vi "reward_behavior_michelle_visjitter_conswin_entice.vi"() -> ()   [LabVIEW 2019]
doc: "The myRIO Project template acquires acceleration data from the onboard accelerometer and displays the changes of acceleration values in a waveform chart."
uses:
  <vilib>/Analysis/Matrix/Datatypes/RealMatrix.ctl
  <vilib>/myRIO/Common/Instrument Driver Framework/myRIO v1.0/Encoder/typedefs/Encoder Signal Mode.ctl
  <vilib>/myRIO/Instrument Drivers/Onboard IO/Encoder/typedefs/Encoder Reference.ctl
  <vilib>/myRIO/Common/Instrument Driver Framework/Utilities/typedefs/myRIO Generic Hardware Reference.ctl
  <vilib>/myRIO/Common/Instrument Driver Framework/Utilities/typedefs/Hardware Version Enum.ctl
  <vilib>/myRIO/Common/Instrument Driver Framework/Utilities/typedefs/myRIO v1.0 Reference.ctl
  <vilib>/myRIO/Common/Instrument Driver Framework/Utilities/typedefs/Generic FPGA Reference.ctl
  <vilib>/myRIO/Common/Instrument Driver Framework/myRIO v1.0/Encoder/typedefs/Encoder Channels Enum.ctl
  <vilib>/myRIO/Common/Instrument Driver Framework/myRIO v1.0/Encoder/typedefs/Encoder Configuration v1.0.ctl
  <vilib>/userdefined/High Color/nirio_resource_hc.ctl
  <vilib>/myRIO/Instrument Drivers/Onboard IO/DIO/typedefs/DIO Reference.ctl
  <vilib>/myRIO/Common/Instrument Driver Framework/myRIO v1.0/DIO/typedefs/DIO Channels List.ctl
  <vilib>/myRIO/Common/Instrument Driver Framework/myRIO v1.0/DIO/typedefs/DIO Channels Enum.ctl
  <vilib>/myRIO/Common/Instrument Driver Framework/Utilities/vis/Is FPGA Ref Available.vi
  <vilib>/myRIO/Common/Instrument Driver Framework/myRIO v1.0/Encoder/vis/myRIO v1.1 Open Encoder.vi
  <vilib>/myRIO/Instrument Drivers/Onboard IO/Encoder/vis/Read.vi
  <vilib>/myRIO/Common/Instrument Driver Framework/myRIO v1.0/DIO/vis/myRIO v1.1 Open DIO.vi
  <vilib>/myRIO/Instrument Drivers/Onboard IO/DIO/vis/Write.vi
  <vilib>/myRIO/Instrument Drivers/Onboard IO/DIO/vis/Read.vi
  <vilib>/myRIO/Common/Instrument Driver Framework/Utilities/vis/Validate Channels.vi
  <vilib>/myRIO/Common/Instrument Driver Framework/myRIO v1.0/Encoder/vis/myRIO v1.0 Reserve Encoder.vi
  <vilib>/myRIO/Common/Instrument Driver Framework/myRIO v1.0/DIO/vis/myRIO v1.0 Reserve DIO.vi
  <vilib>/myRIO/Common/Instrument Driver Framework/myRIO v1.0/Encoder/vis/myRIO v1.0 Build MUX Configuration Encoder.vi
  <vilib>/myRIO/Common/Instrument Driver Framework/myRIO v1.0/Resource Manager/vis/myRIO v1.0 Reserve Channel List.vi
  <vilib>/myRIO/Common/Instrument Driver Framework/myRIO v1.0/DIO/vis/myRIO v1.0 Build MUX Configuration DIO.vi
  <vilib>/myRIO/Common/Instrument Driver Framework/myRIO v1.0/Resource Manager/vis/myRIO v1.0 Create Configuration List.vi
  <vilib>/myRIO/Common/Instrument Driver Framework/myRIO v1.0/Resource Manager/vis/myRIO v1.0 Reserve Channel.vi
  <vilib>/myRIO/Common/Instrument Driver Framework/myRIO v1.0/Resource Manager/vis/myRIO v1.0 Unreserve Channel.vi
  <vilib>/myRIO/Common/Instrument Driver Framework/myRIO v1.0/Resource Manager/vis/myRIO v1.0 Build Mutex Name.vi
  <vilib>/Utility/VariantDataType/GetNumericInfo.vi
  <vilib>/Utility/error.llb/Error Cluster From Error Code.vi
  <vilib>/myRIO/Common/Instrument Driver Framework/myRIO v1.0/myRIO v1.1 Open.vi
  <vilib>/myRIO/Common/Instrument Driver Framework/Utilities/vis/IO Manager.vi
  <vilib>/myRIO/Common/Instrument Driver Framework/Utilities/vis/Configuration Manager.vi
  <vilib>/myRIO/Common/Instrument Driver Framework/myRIO v1.0/Resource Manager/vis/myRIO v1.0 Configure IO.vi
  <vilib>/myRIO/Common/Instrument Driver Framework/myRIO v1.0/myRIO v1.0 Close.vi
  <vilib>/myRIO/Common/Instrument Driver Framework/myRIO v1.0/Encoder/vis/myRIO v1.0 Configure Encoder.vi
  <vilib>/myRIO/Common/Instrument Driver Framework/myRIO v1.0/Encoder/vis/myRIO v1.0 Read Encoder.vi
  <vilib>/myRIO/Common/Instrument Driver Framework/myRIO v1.0/DIO/vis/myRIO v1.0 Read DIO.vi
  <vilib>/myRIO/Common/Instrument Driver Framework/myRIO v1.0/DIO/vis/myRIO v1.0 Write DIO.vi
  <vilib>/myRIO/Express VI/Onboard IO/Encoder/Encoder Express VI.xnode
  <vilib>/myRIO/Instrument Drivers/Onboard IO/Encoder/vis/myRIO Encoder Open.xnode
  <vilib>/myRIO/Express VI/Onboard IO/DI/DI Express VI.xnode
  <vilib>/myRIO/Instrument Drivers/Onboard IO/DIO/vis/myRIO DIO Open.xnode
  <vilib>/myRIO/Express VI/Onboard IO/DO/DO Express VI.xnode
  <vilib>/myRIO/Instrument Drivers/Onboard IO/Encoder/Encoder.lvlib
  <vilib>/myRIO/Instrument Drivers/Onboard IO/DIO/DIO.lvlib
  <vilib>/Analysis/Matrix/NI_Matrix.lvlib
panel:
  out "Enticements":i32
  in  "Entice":bool
  out "Misses":i32
  out "GoAhead":bool
  out "TimeOutDuration":i32
  out "ActiveTime":dbl
  out "ConsumptionGo":bool=TRUE
  out "Consumption_Period":i32
  out "Watch_Display":bool=TRUE
  in  "Give reward":bool
  out "Timings":dbl[](array[numeric])
  out "ISI":dbl
  out "ISI start time":dbl
  out "Time_out":bool=TRUE
  out "Time since lick":dbl
  out "Time of last lick":dbl
  out "Rewarded trials":dbl[](array[numeric])
  out "Rewards":u16
  out "Active Trial":bool
  out "Array temp2":T1
  out "Stimuli Loaded":bool
  out "Stim_ID":dbl[](array[numeric])
  out "Reward_mat":dbl[](array[numeric])
  out "Reward":bool=TRUE
  out "Frame clock":i32
  out "Licks":u32
  out "Lick":bool
  out "Time":dbl
  out "Stop":bool
  in  "Frames to collect":u32
  out "Overflow?":bool
  out "Counter Value":i32
  out "Velocity":dbl
  out "Velocity Plot":dbl[](graph)
  out "Velocity array":dbl[](array[numeric])
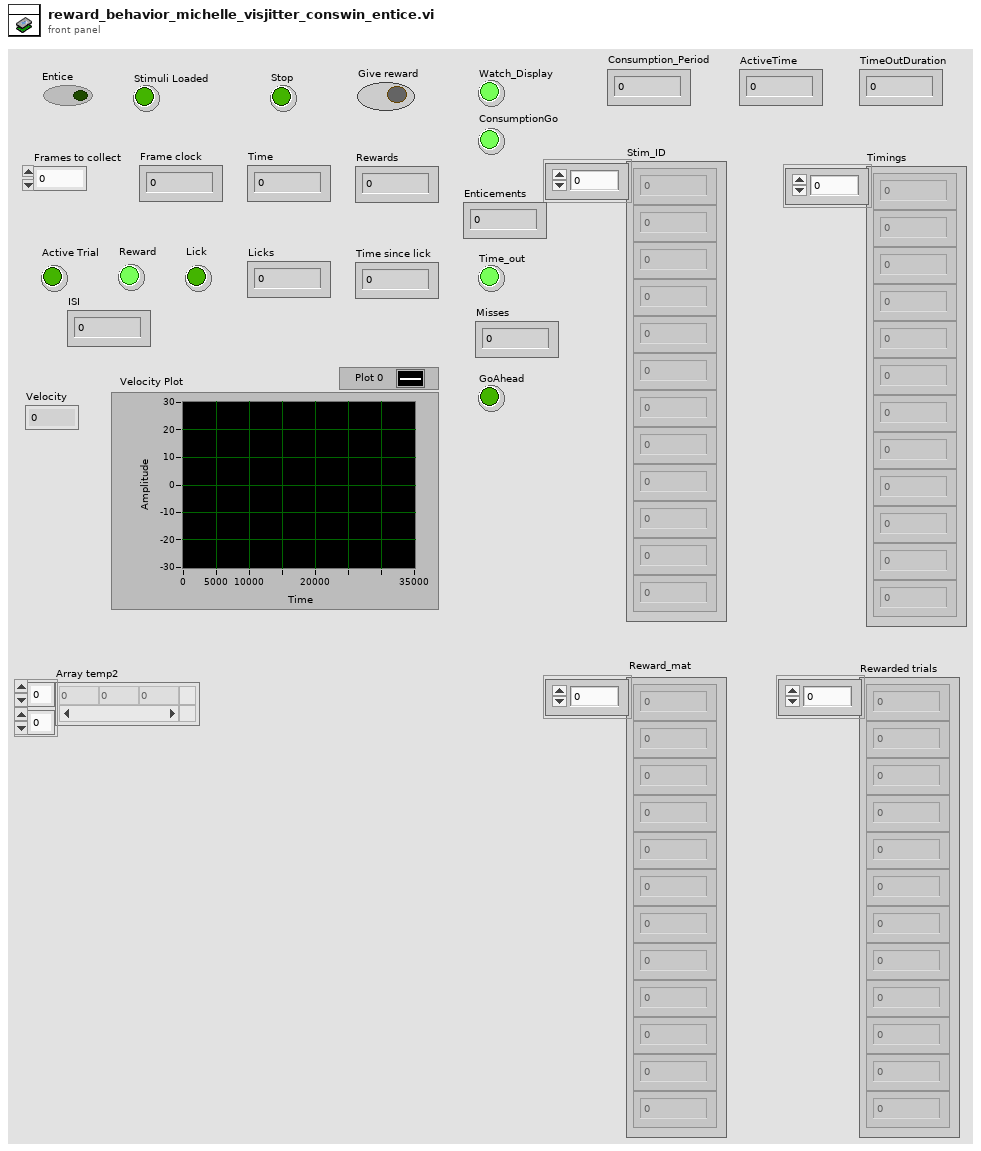
[diagram p1: front panel]
types:
  T1 = typedef "NI_Matrix.lvlib/RealMatrix.ctl" = dbl[][]
  T2 = typedef "Encoder.lvlib/Encoder Reference.ctl" = cluster{"myRIO Reference":T3, "Encoder Channels Enum":T7}
  T3 = typedef "myRIO Generic Hardware Reference.ctl" = cluster{"myRIO Model":T4, "myRIO Hardware Reference":T5}
  T4 = typedef "Hardware Version Enum.ctl" = enum16{"Unknown", "myRIO-1900", "myRIO-1950", "roboRIO", "NI ELVIS RIO CM", "ELVIS III"}
  T5 = typedef "myRIO v1.0 Reference.ctl" = cluster{"Generic FPGA Reference":T6, "Allow multiple opens":bool}
  T6 = typedef "Generic FPGA Reference.ctl" = refnum<k20>
  T7 = typedef "Encoder Channels Enum.ctl" = enum16{"Not Connected", "C/ENC0", "C/ENC1", "A/ENC", "A/ENC0", "A/ENC1", "A/ENC2", "A/ENC3", "A/ENC4", "A/ENC5", "A/ENC6", "A/ENC7", "A/ENC8", "A/ENC9", "B/ENC", "B/ENC0", "B/ENC1", "B/ENC2", "B/ENC3", "B/ENC4", "B/ENC5", "B/ENC6", "B/ENC7", "B/ENC8", "B/ENC9", "DIO/ENC0", "DIO/ENC1", "DIO/ENC2", "DIO/ENC3", "DIO/ENC4"}
  T8 = typedef "Encoder Signal Mode.ctl" = enum16{"Quadrature phase signal", "Step and direction signal"}
  T9 = typedef "nirio_resource_hc.ctl" = tag
  T10 = typedef "DIO.lvlib/DIO Reference.ctl" = cluster{"myRIO Reference":T3, "DIO Channels List":T11}
  T11 = typedef "DIO Channels List.ctl" = T12[]
  T12 = typedef "DIO Channels Enum.ctl" = enum16{"Not Connected", "C/DIO0", "C/DIO1", "C/DIO2", "C/DIO3", "C/DIO4", "C/DIO5", "C/DIO6", "C/DIO7", "A/DIO0", "A/DIO1", "A/DIO2", "A/DIO3", "A/DIO4", "A/DIO5", "A/DIO6", "A/DIO7", "A/DIO8", "A/DIO9", "A/DIO10", "A/DIO11", "A/DIO12", "A/DIO13", "A/DIO14", "A/DIO15", "A/DIO16", "A/DIO17", "A/DIO18", "A/DIO19", "B/DIO0", "B/DIO1", "B/DIO2", "B/DIO3", "B/DIO4", "B/DIO5", "B/DIO6", "B/DIO7", "B/DIO8", "B/DIO9", "B/DIO10", "B/DIO11", "B/DIO12", "B/DIO13", "B/DIO14", "B/DIO15", "B/DIO16", "B/DIO17", "B/DIO18", "B/DIO19", "LED0", "LED1", "LED2", "LED3", "Button0", "DIO/DIO0", "DIO/DIO1", "DIO/DIO2", "DIO/DIO3", "DIO/DIO4", "DIO/DIO5", "DIO/DIO6", "DIO/DIO7", "DIO/DIO8", "DIO/DIO9", "SPI/CS0", "SPI/CS1", "SPI/CS2", "SPI/CS3", "LED RADIO (Green)", "LED RADIO (Red)", "LED COMM (Green)", "LED COMM (Red)", "LED MODE (Green)", "LED MODE (Red)"}
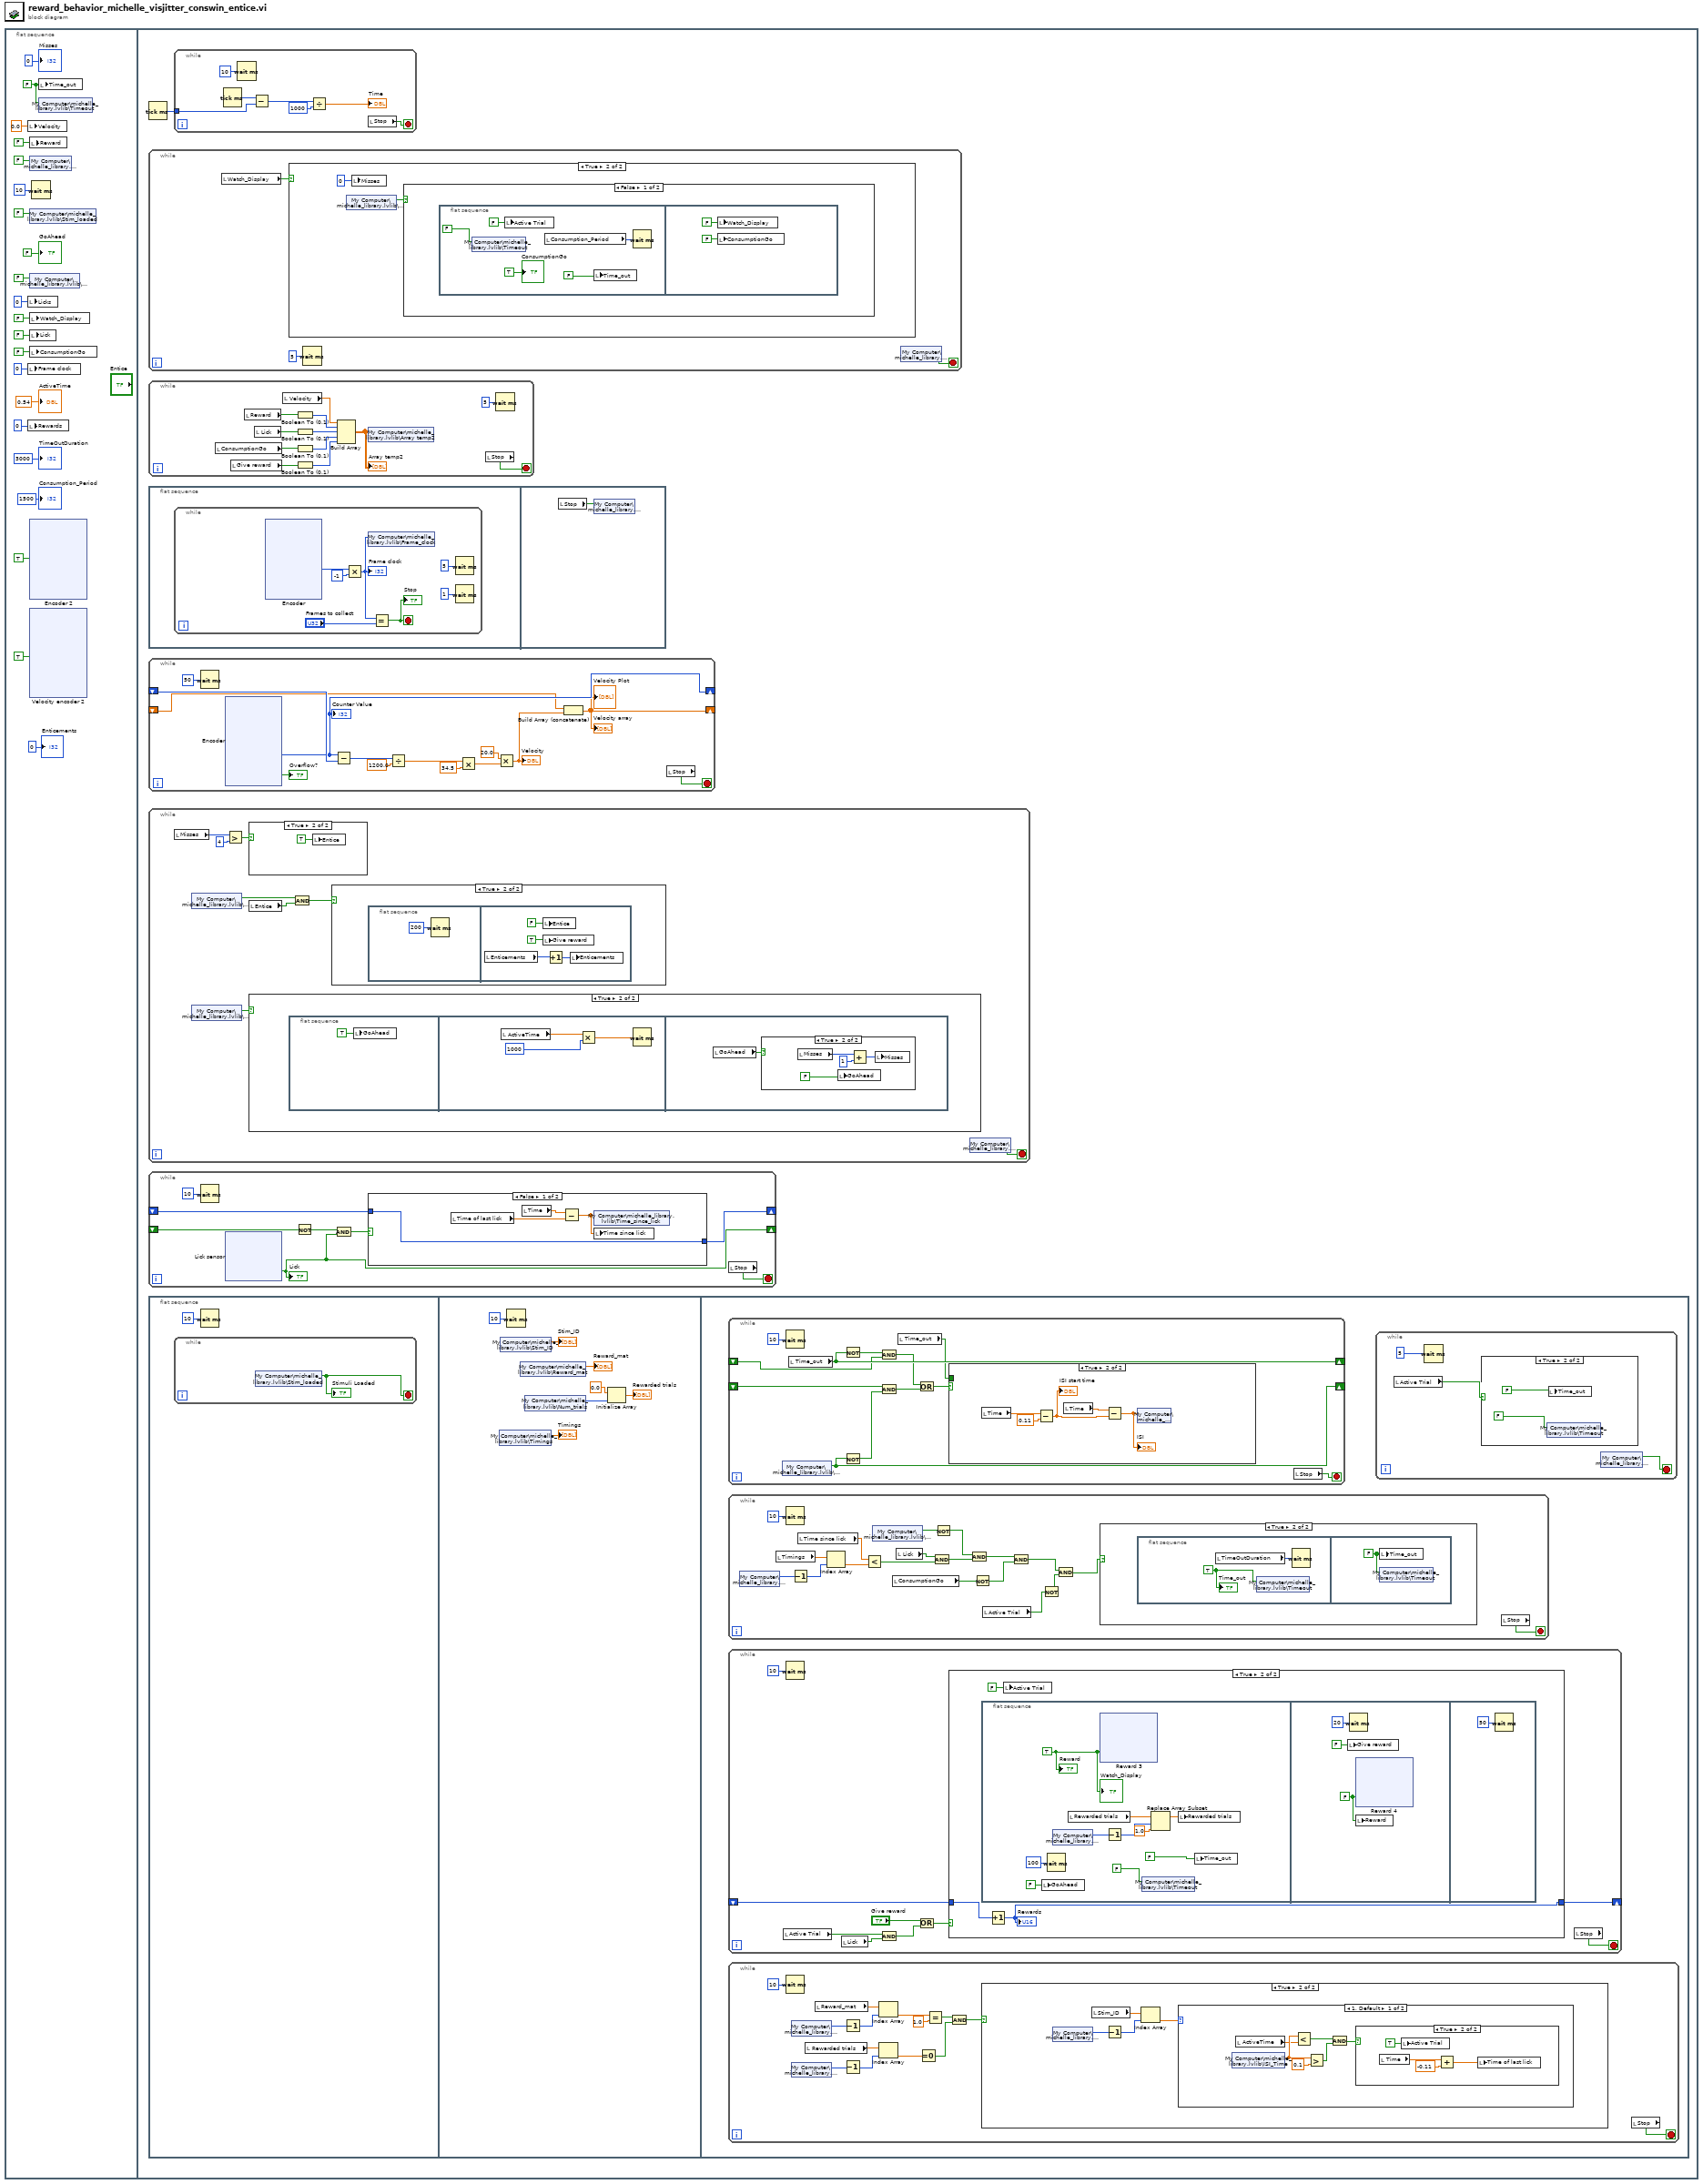
[diagram p0: block diagram]
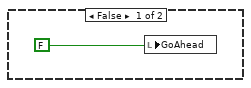
[diagram p4: hidden frame]
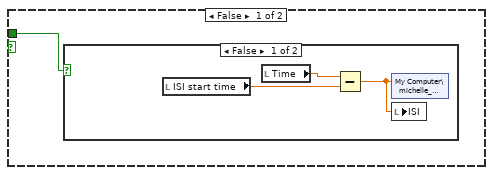
[diagram p10: hidden frame]
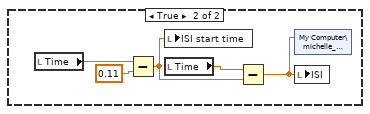
[diagram p11: hidden frame]
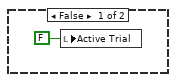
[diagram p12: hidden frame]
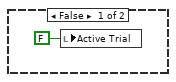
[diagram p13: hidden frame]
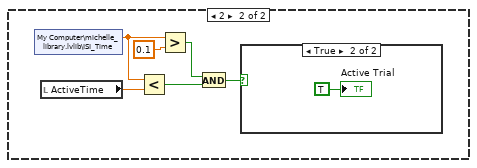
[diagram p14: hidden frame]
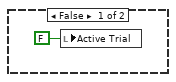
[diagram p15: hidden frame]
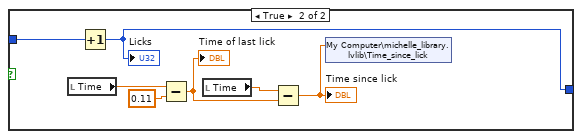
[diagram p17: hidden frame]
diagram:
  n1 = flat-sequence {
    frame #0 {
      w9 = FALSE ("Time_out")
      n2 = local write "Velocity"(0.0 ("Velocity")) -> ()
      n3 = local write "Licks"(u32 0 ("Licks")) -> ()
      n4 = local write "Frame clock"(u32 0 ("Frames")) -> ()
      n5 = local write "Rewards"(u16 0 ("Rewards")) -> ()
      n6 = local write "Reward"(FALSE ("Give reward")) -> ()
      n7 = shared-variable "My Computer\\michelle_library.lvlib\\Stop"(FALSE ("Stop")) -> ()  [unwired: 1 in, 1 out]
      n8 = shared-variable "My Computer\\michelle_library.lvlib\\Stim_loaded"(FALSE ("Stim_loaded")) -> ()  [unwired: 1 in, 1 out]
      n9 = shared-variable "My Computer\\michelle_library.lvlib\\Display"(FALSE ("Display")) -> ()  [unwired: 1 in, 1 out]
      n10 = local write "Watch_Display"(FALSE ("Watch_Display")) -> ()
      n11 = local write "Lick"(FALSE ("Lick")) -> ()
      n12 = local write "ConsumptionGo"(FALSE ("ConsumptionGo")) -> ()
      n13 = xnode "Encoder 2"("Reset Counter"=TRUE) -> ()  [unwired: 1 in, 4 out]
      n14 = xnode "Velocity encoder 2"("Reset Counter"=TRUE) -> ()  [unwired: 1 in, 4 out]
      n15 = Wait (ms)(milliseconds to wait=u32 10) -> ()  [unwired: 1 out]
      n16 = local write "Time_out"(w9) -> ()
      n17 = shared-variable "My Computer\\michelle_library.lvlib\\Timeout"(w9) -> ()  [unwired: 1 in, 1 out]
      "Consumption_Period" <- 1500
      "ActiveTime" <- 0.54
      "TimeOutDuration" <- 3000
      "GoAhead" <- FALSE
      "Misses" <- 0
      "Enticements" <- 0
    }
    frame #1 {
      n18 = Tick Count (ms)() -> (millisecond timer value=w114:u32)
      n19 = while {
        stop <- w141 stop-if-true
        n20 = local read "Watch_Display"() -> (w140:bool)
        n21 = case shown="True" w140 {
          frame False {
          }
          frame True {
            n22 = shared-variable "My Computer\\michelle_library.lvlib\\Display"() -> (w143:bool)  [unwired: 1 in, 1 out]
            n23 = local write "Misses"(0) -> ()
            n24 = case shown="False" w143 {
              frame False {
                n25 = flat-sequence {
                  frame #0 {
                    n26 = shared-variable "My Computer\\michelle_library.lvlib\\Timeout"(FALSE) -> ()  [unwired: 1 in, 1 out]
                    n27 = local write "Active Trial"(FALSE) -> ()
                    n28 = local read "Consumption_Period"() -> (w148:i32)
                    n29 = local write "Time_out"(FALSE) -> ()
                    n30 = Wait (ms)(milliseconds to wait=w148) -> ()  [unwired: 1 out]
                    "ConsumptionGo" <- TRUE
                  }
                  frame #1 {
                    n31 = local write "Watch_Display"(FALSE ("Watch_Display")) -> ()
                    n32 = local write "ConsumptionGo"(FALSE ("ConsumptionGo")) -> ()
                  }
                }
              }
              frame True {
              }
            }
          }
        }
        n33 = Wait (ms)(milliseconds to wait=u32 5) -> ()  [unwired: 1 out]
        n34 = shared-variable "My Computer\\michelle_library.lvlib\\Stop"() -> (w141:bool)  [unwired: 1 in, 1 out]
      }
      n35 = while {
        stop <- w156 stop-if-true
        n36 = local read "ConsumptionGo"() -> (w154:bool)
        n37 = local read "Give reward"() -> (w153:bool)
        n38 = local read "Reward"() -> (w161:bool)
        n39 = local read "Lick"() -> (w162:bool)
        n40 = local read "Velocity"() -> (w160:dbl)
        n41 = Boolean To (0,1)(Boolean=w161) -> (0, 1=w159:i16)
        n42 = Boolean To (0,1)(Boolean=w162) -> (0, 1=w158:i16)
        n43 = Boolean To (0,1)(Boolean=w154) -> (0, 1=w152:i16)
        n44 = Boolean To (0,1)(Boolean=w153) -> (0, 1=w151:i16)
        n45 = Build Array(w160, w159, w158, w152, w151) -> (w155:T1)
        "Array temp2" <- w155
        n46 = shared-variable "My Computer\\michelle_library.lvlib\\Array temp2"(w155) -> ()  [unwired: 1 in, 1 out]
        n47 = local read "Stop"() -> (w156:bool)
        n48 = Wait (ms)(milliseconds to wait=u32 5) -> ()  [unwired: 1 out]
      }
      n49 = flat-sequence {
        frame #0 {
          n50 = while {
            stop <- w361 stop-if-true
            n51 = xnode "Encoder"() -> ("Counter Value"=w365:i32)  [unwired: 2 in, 3 out]
            n52 = Multiply(x=w365, y=-1) -> (x*y=w360:i32)
            "Frame clock" <- w360
            n53 = shared-variable "My Computer\\michelle_library.lvlib\\Frame_clock"(w360) -> ()  [unwired: 1 in, 1 out]
            n54 = Equal?(x=w360, y="Frames to collect") -> (x = y?=w361:bool)
            "Stop" <- w361
            n55 = Wait (ms)(milliseconds to wait=u32 5) -> ()  [unwired: 1 out]
            n56 = Wait (ms)(milliseconds to wait=u32 1) -> ()  [unwired: 1 out]
          }
        }
        frame #1 {
          n57 = local read "Stop"() -> (w413:bool)
          n58 = shared-variable "My Computer\\michelle_library.lvlib\\Stop"(w413) -> ()  [unwired: 1 in, 1 out]
        }
      }
      n59 = while {
        shift-right: [w478] -> _
        shift-left: _ -> [w479]
        shift-right: [w470] -> _
        shift-left: _ -> [w469]
        stop <- w468 stop-if-true
        n60 = Wait (ms)(milliseconds to wait=u32 50) -> ()  [unwired: 1 out]
        n61 = xnode "Encoder"() -> ("Counter Value"=w478:i32, "Overflow?"=→"Overflow?":bool)  [unwired: 2 in, 2 out]
        "Counter Value" <- w478
        n62 = Subtract(x=w478, y=w479) -> (x-y=w471:i32)
        n63 = Divide(x=w471, y=1200.0 ("600")) -> (x/y=w476:dbl)
        n64 = Multiply(x=w476, y=34.5) -> (x*y=w474:dbl)
        n65 = Multiply(x=20.0, y=w474) -> (x*y=w472:dbl)
        "Velocity" <- w472
        n66 = Build Array (concatenate)(w469, w472) -> (w470:dbl[])
        "Velocity Plot" <- w470
        "Velocity array" <- w470
        n67 = local read "Stop"() -> (w468:bool)
      }
      n68 = while {
        stop <- w122 stop-if-true
        n69 = local read "Misses"() -> (w120:i32)
        n70 = shared-variable "My Computer\\michelle_library.lvlib\\Display"() -> (w116:bool)  [unwired: 1 in, 1 out]
        n71 = shared-variable "My Computer\\michelle_library.lvlib\\Display"() -> (w121:bool)  [unwired: 1 in, 1 out]
        n72 = Greater?(x=w120, y=4) -> (0:w118:bool)
        n73 = case shown="True" w118 {
          frame False {
          }
          frame True {
            n74 = local write "Entice"(TRUE) -> ()
          }
        }
        n75 = local read "Entice"() -> (w115:bool)
        n76 = case shown="True" w121 {
          frame False {
            n77 = local write "GoAhead"(FALSE) -> ()
          }
          frame True {
            n78 = flat-sequence {
              frame #0 {
                n79 = local write "GoAhead"(TRUE) -> ()
              }
              frame #1 {
                n80 = local read "ActiveTime"() -> (w133:dbl)
                n81 = Multiply(x=w133, y=1000) -> (x*y=w131:dbl)
                n82 = Wait (ms)(milliseconds to wait=w131) -> ()  [unwired: 1 out]
              }
              frame #2 {
                n83 = local read "GoAhead"() -> (w134:bool)
                n84 = case shown="True" w134 {
                  frame False {
                  }
                  frame True {
                    n85 = local read "Misses"() -> (w138:i32)
                    n86 = local write "GoAhead"(FALSE) -> ()
                    n87 = Add(x=w138, y=1) -> (x+y=w136:i32)
                    n88 = local write "Misses"(w136) -> ()
                  }
                }
              }
            }
          }
        }
        n89 = And(x=w116, y=w115) -> (x .and. y?=w117:bool)
        n90 = case shown="True" w117 {
          frame False {
          }
          frame True {
            n91 = flat-sequence {
              frame #0 {
                n92 = Wait (ms)(milliseconds to wait=200) -> ()  [unwired: 1 out]
              }
              frame #1 {
                n93 = local read "Enticements"() -> (w125:i32)
                n94 = local write "Entice"(FALSE) -> ()
                n95 = local write "Give reward"(TRUE) -> ()
                n96 = Increment(x=w125) -> (x+1=w124:i32)
                n97 = local write "Enticements"(w124) -> ()
              }
            }
          }
        }
        n98 = shared-variable "My Computer\\michelle_library.lvlib\\Stop"() -> (w122:bool)  [unwired: 1 in, 1 out]
      }
      n99 = while {
        shift-right: [w420] -> _
        shift-left: _ -> [w419]
        shift-right: [w414] -> _
        shift-left: _ -> [w417]
        stop <- w418 stop-if-true
        n100 = Wait (ms)(milliseconds to wait=u32 10) -> ()  [unwired: 1 out]
        n101 = xnode "Lick sensor"() -> ("C/DIO1 (DIO1)"=w414:bool)  [unwired: 1 in, 1 out]
        "Lick" <- w414
        n102 = Not(x=w417) -> (.not. x?=w416:bool)
        n103 = And(x=w416, y=w414) -> (x .and. y?=w415:bool)
        n104 = case shown="False" w415 {
          tunnel: [w425 w432] -> w420
          tunnel: w419 -> [w425 w431]
          frame False {
            n105 = local read "Time of last lick"() -> (w423:dbl)
            n106 = local read "Time"() -> (w424:dbl)
            n107 = Subtract(x=w424, y=w423) -> (x-y=w422:dbl)
            n108 = shared-variable "My Computer\\michelle_library.lvlib\\Time_since_lick"(w422) -> ()  [unwired: 1 in, 1 out]
            n109 = local write "Time since lick"(w422) -> ()
          }
          frame True {
            n110 = local read "Time"() -> (w428:dbl)
            n111 = Increment(x=w431) -> (x+1=w432:u32)
            "Licks" <- w432
            n112 = Subtract(x=w428, y=0.11) -> (x-y=w426:dbl)
            "Time of last lick" <- w426
            n113 = local read "Time"() -> (w430:dbl)
            n114 = Subtract(x=w430, y=w426) -> (x-y=w429:dbl)
            "Time since lick" <- w429
            n115 = shared-variable "My Computer\\michelle_library.lvlib\\Time_since_lick"(w429) -> ()  [unwired: 1 in, 1 out]
          }
        }
        n116 = local read "Stop"() -> (w418:bool)
      }
      n117 = flat-sequence {
        frame #0 {
          n118 = while {
            stop <- w164 stop-if-true
            n119 = shared-variable "My Computer\\michelle_library.lvlib\\Stim_loaded"() -> (w164:bool)  [unwired: 1 in, 1 out]
            "Stimuli Loaded" <- w164
          }
          n120 = Wait (ms)(milliseconds to wait=u32 10) -> ()  [unwired: 1 out]
        }
        frame #1 {
          n121 = shared-variable "My Computer\\michelle_library.lvlib\\Timings"() -> (→"Timings":dbl[])  [unwired: 1 in, 1 out]
          n122 = shared-variable "My Computer\\michelle_library.lvlib\\Stim_ID"() -> (→"Stim_ID":dbl[])  [unwired: 1 in, 1 out]
          n123 = Wait (ms)(milliseconds to wait=u32 10) -> ()  [unwired: 1 out]
          n124 = shared-variable "My Computer\\michelle_library.lvlib\\Reward_mat"() -> (→"Reward_mat":dbl[])  [unwired: 1 in, 1 out]
          n125 = shared-variable "My Computer\\michelle_library.lvlib\\Num_trials"() -> (w168:u32)  [unwired: 1 in, 1 out]
          n126 = Initialize Array(0.0 ("element"), w168) -> (→"Rewarded trials":dbl[])
        }
        frame #2 {
          n127 = while {
            shift-right: [w209] -> _
            shift-left: _ -> [w207]
            shift-right: [w205] -> _
            shift-left: _ -> [w204]
            stop <- w210 stop-if-true
            n128 = shared-variable "My Computer\\michelle_library.lvlib\\Display"() -> (w205:bool)  [unwired: 1 in, 1 out]
            n129 = Wait (ms)(milliseconds to wait=u32 10) -> ()  [unwired: 1 out]
            n130 = local read "Time_out"() -> (w209:bool)
            n131 = Not(x=w209) -> (.not. x?=w208:bool)
            n132 = Not(x=w205) -> (.not. x?=w203:bool)
            n133 = And(x=w208, y=w207) -> (x .and. y?=w202:bool)
            n134 = And(x=w204, y=w203) -> (x .and. y?=w201:bool)
            n135 = local read "Time_out"() -> (w206:bool)
            n136 = Or(x=w202, y=w201) -> (x .or. y?=w200:bool)
            n137 = case shown="True" w200 {
              tunnel: w206 -> [w211 _]
              frame False {
                n138 = case shown="False" w211 {
                  frame False {
                    n139 = local read "ISI start time"() -> (w214:dbl)
                    n140 = local read "Time"() -> (w213:dbl)
                    n141 = Subtract(x=w213, y=w214) -> (x-y=w212:dbl)
                    n142 = shared-variable "My Computer\\michelle_library.lvlib\\ISI"(w212) -> ()  [unwired: 1 in, 1 out]
                    n143 = local write "ISI"(w212) -> ()
                  }
                  frame True {
                    n144 = local read "Time"() -> (w219:dbl)
                    n145 = Subtract(x=w219, y=0.11) -> (x-y=w216:dbl)
                    n146 = local write "ISI start time"(w216) -> ()
                    n147 = local read "Time"() -> (w217:dbl)
                    n148 = Subtract(x=w217, y=w216) -> (x-y=w215:dbl)
                    n149 = shared-variable "My Computer\\michelle_library.lvlib\\ISI"(w215) -> ()  [unwired: 1 in, 1 out]
                    n150 = local write "ISI"(w215) -> ()
                  }
                }
              }
              frame True {
                n151 = local read "Time"() -> (w224:dbl)
                n152 = Subtract(x=w224, y=0.11) -> (x-y=w221:dbl)
                "ISI start time" <- w221
                n153 = local read "Time"() -> (w222:dbl)
                n154 = Subtract(x=w222, y=w221) -> (x-y=w220:dbl)
                "ISI" <- w220
                n155 = shared-variable "My Computer\\michelle_library.lvlib\\ISI"(w220) -> ()  [unwired: 1 in, 1 out]
              }
            }
            n156 = local read "Stop"() -> (w210:bool)
          }
          n157 = while {
            stop <- w195 stop-if-true
            n158 = shared-variable "My Computer\\michelle_library.lvlib\\Trial"() -> (w185:u32)  [unwired: 1 in, 1 out]
            n159 = local read "Timings"() -> (w187:dbl[])
            n160 = Wait (ms)(milliseconds to wait=u32 10) -> ()  [unwired: 1 out]
            n161 = Decrement(x=w185) -> (x-1=w184:u32)
            n162 = local read "Time since lick"() -> (w194:dbl)
            n163 = Index Array(array=w187, index=w184) -> (element=w186:dbl)
            n164 = Less?(x=w194, y=w186) -> (x < y?=w193:bool)
            n165 = shared-variable "My Computer\\michelle_library.lvlib\\Display"() -> (w190:bool)  [unwired: 1 in, 1 out]
            n166 = local read "ConsumptionGo"() -> (w182:bool)
            n167 = local read "Lick"() -> (w192:bool)
            n168 = And(x=w192, y=w193) -> (x .and. y?=w188:bool)
            n169 = Not(x=w190) -> (.not. x?=w189:bool)
            n170 = And(x=w189, y=w188) -> (x .and. y?=w181:bool)
            n171 = Not(x=w182) -> (.not. x?=w183:bool)
            n172 = local read "Active Trial"() -> (w177:bool)
            n173 = And(x=w181, y=w183) -> (x .and. y?=w179:bool)
            n174 = Not(x=w177) -> (.not. x?=w180:bool)
            n175 = And(x=w179, y=w180) -> (x .and. y?=w178:bool)
            n176 = case shown="True" w178 {
              frame False {
              }
              frame True {
                n177 = flat-sequence {
                  frame #0 {
                    w197 = TRUE
                    n178 = local read "TimeOutDuration"() -> (w196:i32)
                    n179 = shared-variable "My Computer\\michelle_library.lvlib\\Timeout"(w197) -> ()  [unwired: 1 in, 1 out]
                    n180 = Wait (ms)(milliseconds to wait=w196) -> ()  [unwired: 1 out]
                    "Time_out" <- w197
                  }
                  frame #1 {
                    w198 = FALSE ("Timeout")
                    n181 = local write "Time_out"(w198) -> ()
                    n182 = shared-variable "My Computer\\michelle_library.lvlib\\Timeout"(w198) -> ()  [unwired: 1 in, 1 out]
                  }
                }
              }
            }
            n183 = local read "Stop"() -> (w195:bool)
          }
          n184 = while {
            shift-right: [w269] -> _
            shift-left: _ -> [w268]
            stop <- w271 stop-if-true
            n185 = local read "Active Trial"() -> (w266:bool)
            n186 = Wait (ms)(milliseconds to wait=u32 10) -> ()  [unwired: 1 out]
            n187 = local read "Lick"() -> (w267:bool)
            n188 = And(x=w266, y=w267) -> (x .and. y?=w265:bool)
            n189 = Or(x="Give reward", y=w265) -> (x .or. y?=w264:bool)
            n190 = case shown="True" w264 {
              tunnel: [w272 w275] -> w269
              tunnel: w268 -> [w272 w274]
              frame False {
              }
              frame True {
                n191 = flat-sequence {
                  frame #0 {
                    w284 = TRUE ("C/DIO0 (DIO0)")
                    n192 = local write "GoAhead"(FALSE) -> ()
                    n193 = Wait (ms)(milliseconds to wait=u32 100) -> ()  [unwired: 1 out]
                    n194 = shared-variable "My Computer\\michelle_library.lvlib\\Trial"() -> (w283:u32)  [unwired: 1 in, 1 out]
                    n195 = local read "Rewarded trials"() -> (w281:dbl[])
                    n196 = xnode "Reward 3"("C/DIO0 (DIO0)"=w284) -> ()  [unwired: 1 in, 1 out]
                    n197 = Decrement(x=w283) -> (x-1=w282:u32)
                    n198 = shared-variable "My Computer\\michelle_library.lvlib\\Timeout"(FALSE) -> ()  [unwired: 1 in, 1 out]
                    n199 = Replace Array Subset(array=w281, new element=1.0 ("new element/subarray"), index=w282) -> (w279:dbl[])
                    n200 = local write "Rewarded trials"(w279) -> ()
                    n201 = local write "Time_out"(FALSE) -> ()
                    "Reward" <- w284
                    "Watch_Display" <- w284
                  }
                  frame #1 {
                    w323 = FALSE ("C/DIO0 (DIO0)")
                    n202 = local write "Give reward"(FALSE ("Give reward")) -> ()
                    n203 = Wait (ms)(milliseconds to wait=u32 20) -> ()  [unwired: 1 out]
                    n204 = xnode "Reward 4"("C/DIO0 (DIO0)"=w323) -> ()  [unwired: 1 in, 1 out]
                    n205 = local write "Reward"(w323) -> ()
                  }
                  frame #2 {
                    n206 = Wait (ms)(milliseconds to wait=u32 50) -> ()  [unwired: 1 out]
                  }
                }
                n207 = Increment(x=w274) -> (x+1=w275:u16)
                "Rewards" <- w275
                n208 = local write "Active Trial"(FALSE ("Active Trial")) -> ()
              }
            }
            n209 = local read "Stop"() -> (w271:bool)
          }
          n210 = while {
            stop <- w238 stop-if-true
            n211 = Wait (ms)(milliseconds to wait=u32 10) -> ()  [unwired: 1 out]
            n212 = shared-variable "My Computer\\michelle_library.lvlib\\Trial"() -> (w234:u32)  [unwired: 1 in, 1 out]
            n213 = shared-variable "My Computer\\michelle_library.lvlib\\Trial"() -> (w230:u32)  [unwired: 1 in, 1 out]
            n214 = local read "Rewarded trials"() -> (w231:dbl[])
            n215 = local read "Reward_mat"() -> (w233:dbl[])
            n216 = Decrement(x=w234) -> (x-1=w235:u32)
            n217 = Decrement(x=w230) -> (x-1=w229:u32)
            n218 = Index Array(array=w233, index=w235) -> (element=w236:dbl)
            n219 = Index Array(array=w231, index=w229) -> (element=w228:dbl)
            n220 = Equal To 0?(x=w228) -> (x = 0?=w227:bool)
            n221 = Equal?(x=w236, y=1.0) -> (x = y?=w226:bool)
            n222 = And(x=w226, y=w227) -> (x .and. y?=w225:bool)
            n223 = case shown="True" w225 {
              frame False {
                n224 = local write "Active Trial"(FALSE ("Active_trial")) -> ()
              }
              frame True {
                n225 = shared-variable "My Computer\\michelle_library.lvlib\\Trial"() -> (w241:u32)  [unwired: 1 in, 1 out]
                n226 = local read "Stim_ID"() -> (w243:dbl[])
                n227 = Decrement(x=w241) -> (x-1=w242:u32)
                n228 = Index Array(array=w243, index=w242) -> (element=w240:dbl)
                n229 = case shown="1, Default" w240 {
                  frame 1, Default {
                    n230 = shared-variable "My Computer\\michelle_library.lvlib\\ISI_Time"() -> (w249:dbl)  [unwired: 1 in, 1 out]
                    n231 = local read "ActiveTime"() -> (w244:dbl)
                    n232 = Less?(x=w249, y=w244) -> (x < y?=w247:bool)
                    n233 = Greater?(x=w249, y=0.1) -> (0:w246:bool)
                    n234 = And(x=w247, y=w246) -> (x .and. y?=w245:bool)
                    n235 = case shown="True" w245 {
                      frame False {
                        n236 = local write "Active Trial"(FALSE ("Active Trial")) -> ()
                      }
                      frame True {
                        n237 = local read "Time"() -> (w253:dbl)
                        n238 = local write "Active Trial"(TRUE ("Active Trial")) -> ()
                        n239 = Add(x=w253, y=-0.11) -> (x+y=w251:dbl)
                        n240 = local write "Time of last lick"(w251) -> ()
                      }
                    }
                  }
                  frame 2 {
                    n241 = shared-variable "My Computer\\michelle_library.lvlib\\ISI_Time"() -> (w259:dbl)  [unwired: 1 in, 1 out]
                    n242 = local read "ActiveTime"() -> (w255:dbl)
                    n243 = Less?(x=w259, y=w255) -> (x < y?=w257:bool)
                    n244 = Greater?(x=w259, y=0.1) -> (0:w258:bool)
                    n245 = And(x=w258, y=w257) -> (x .and. y?=w256:bool)
                    n246 = case shown="True" w256 {
                      frame False {
                        n247 = local write "Active Trial"(FALSE ("Active Trial")) -> ()
                      }
                      frame True {
                        "Active Trial" <- TRUE ("Active Trial")
                      }
                    }
                  }
                }
              }
            }
            n248 = local read "Stop"() -> (w238:bool)
          }
          n249 = while {
            stop <- w174 stop-if-true
            n250 = local read "Active Trial"() -> (w173:bool)
            n251 = Wait (ms)(milliseconds to wait=5) -> ()  [unwired: 1 out]
            n252 = case shown="True" w173 {
              frame False {
              }
              frame True {
                n253 = shared-variable "My Computer\\michelle_library.lvlib\\Timeout"(FALSE) -> ()  [unwired: 1 in, 1 out]
                n254 = local write "Time_out"(FALSE) -> ()
              }
            }
            n255 = shared-variable "My Computer\\michelle_library.lvlib\\Stop"() -> (w174:bool)  [unwired: 1 in, 1 out]
          }
        }
      }
      n256 = while {
        tunnel: w114 -> [w533]
        stop <- w531 stop-if-true
        n257 = Tick Count (ms)() -> (millisecond timer value=w534:u32)
        n258 = Wait (ms)(milliseconds to wait=u32 10) -> ()  [unwired: 1 out]
        n259 = Subtract(x=w534, y=w533) -> (x-y=w530:u32)
        n260 = Divide(x=w530, y=u32 1000) -> (x/y=→"Time":dbl)
        n261 = local read "Stop"() -> (w531:bool)
      }
    }
  }
